vi "Destroy.vi"(11 "TEMPLATE jettl in":refnum<class "TEMPLATE Actor.lvclass">) -> (3 "TEMPLATE jettl out":refnum<class "TEMPLATE Actor.lvclass">)   [LabVIEW 2021, in "_Template.lvlib" / "Templates.lvlib" / "TEMPLATE Actor.lvlib" / "TEMPLATE Actor.lvclass"]
uses:
  TEMPLATE Actor.lvclass
  jettl/jettl/jettl/jettl.lvclass
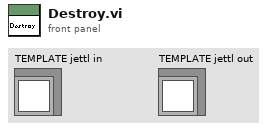
[diagram p1: front panel]
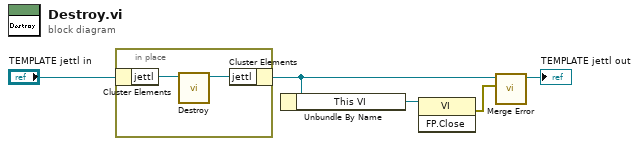
[diagram p0: block diagram]
diagram:
  n1 = in-place {
    n2 = in-place-cluster #1("TEMPLATE jettl in") -> ("jettl"=w7:refnum<class "jettl.lvclass">)
    n3 = call-dynamic "Destroy.vi"("jettl in"=w7) -> ("jettl out"=w6:refnum<class "jettl.lvclass">)  [unwired: 10 in]
    n4 = in-place-cluster #1("jettl"=w6) -> (w2:refnum<class "TEMPLATE Actor.lvclass">)
  }
  n5 = Unbundle By Name(w2) -> ("This VI"=w1:refnum<vi>)
  n6 = invoke class="VI" method="FP.Close"(reference=w1) -> (error out=w4:errorcluster)  [unwired: 2 in, 2 out]
  n7 = call-dynamic "Merge Error.vi"("Error"=w4, "TEMPLATE jettl in"=w2) -> ("TEMPLATE jettl out"=→"TEMPLATE jettl out":refnum<class "TEMPLATE Actor.lvclass">)  [unwired: 9 in]
